vi "Main.vi"() -> ()   [LabVIEW 2020]
panel:
  out "TempF":dbl
  in  "TempC":dbl
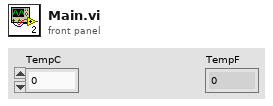
[diagram p1: front panel]
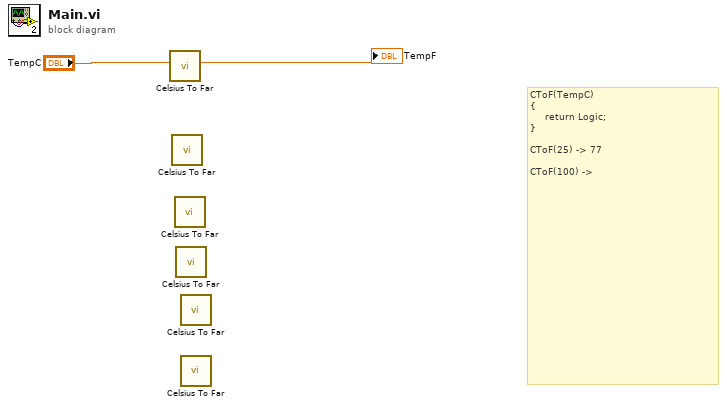
[diagram p0: block diagram]
diagram:
  # "CToF(TempC)\n{\n     return Logic;\n}\n\nCToF(25) -> 77\n\nCToF(100) ->"
  n1 = call "Celsius To Far.vi"("TempC"="TempC") -> ("TempF"=→"TempF":dbl)  [unwired: 10 in]
  n2 = call "Celsius To Far.vi"() -> ()  [unwired: 11 in, 1 out]
  n3 = call "Celsius To Far.vi"() -> ()  [unwired: 11 in, 1 out]
  n4 = call "Celsius To Far.vi"() -> ()  [unwired: 11 in, 1 out]
  n5 = call "Celsius To Far.vi"() -> ()  [unwired: 11 in, 1 out]
  n6 = call "Celsius To Far.vi"() -> ()  [unwired: 11 in, 1 out]
